vi "Create comm references.vi"() -> (0 "error out":errorcluster)   [LabVIEW 2019, in "Shared.lvlib"]
uses:
  Shared.lvlib
  Intertarget communication/Command + data + response cluster.ctl
  Intertarget communication/Status + response + data cluster.ctl
  Data message cluster.ctl
  mmWave data_class/mmWave data.lvclass
  Error event data.ctl
  Comm GV.vi
  Intertarget communication/CommandResponse communication.lvlib
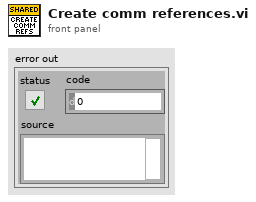
[diagram p1: front panel]
types:
  T1 = typedef "Shared.lvlib/Error event data.ctl" = cluster{"module":string, "info":string, "error":cluster{"Boolean Round":bool, "code":i32, "source":string}}
  T2 = typedef "Shared.lvlib/Data message cluster.ctl" = cluster{"group  ":string, "Data":refnum<class "mmWave data.lvclass">}
  T3 = typedef "CommandResponse communication.lvlib/Command + data + response cluster.ctl" = cluster{"message":string, "parameters":string, "response notifier":refnum<notifier>, "data":variant}
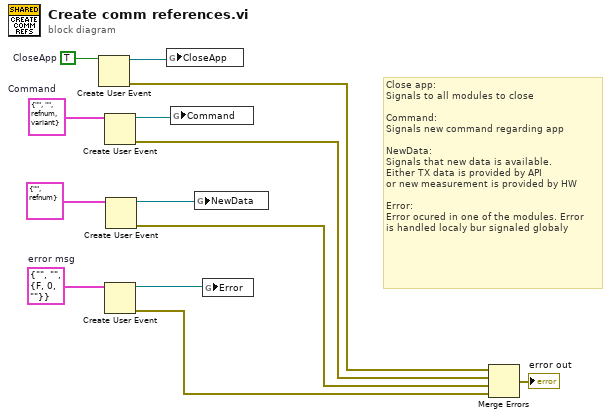
[diagram p0: block diagram]
diagram:
  w10 = T1 {"module"="", "info"="", "error"={"Boolean Round"=FALSE, "code"=0, "source"=""}}  # error msg
  w12 = T3 {"message"="", "parameters"="", "response notifier"=refnum, "data"=variant}  # Command
  w13 = TRUE  # CloseApp
  # "Close app:\nSignals to all modules to close\n\nCommand:\nSignals new command regarding app\n\nNewData:\nSignals that new data is available.\nEither TX data is provided by API\nor new measurement is provided by HW\n\nError:\nError ocured in one of the modules. Error\nis handled localy bur signaled globaly"
  n1 = Create User Event(user event datatype=w13) -> (user event=w4:refnum<user-event>, error out=w9:errorcluster)  [unwired: 1 in]
  n2 = Create User Event(user event datatype=w12) -> (user event=w3:refnum<user-event>, error out=w8:errorcluster)  [unwired: 1 in]
  n3 = Create User Event(user event datatype=w10) -> (user event=w1:refnum<user-event>, error out=w6:errorcluster)  [unwired: 1 in]
  n4 = Create User Event(user event datatype=T2 {"group  "="", "Data"=refnum} ("New data message")) -> (user event=w2:refnum<user-event>, error out=w7:errorcluster)  [unwired: 1 in]
  n5 = global write "Comm GV.vi" "CloseApp"(w4) -> ()
  n6 = global write "Comm GV.vi" "Command"(w3) -> ()
  n7 = global write "Comm GV.vi" "NewData"(w2) -> ()
  n8 = global write "Comm GV.vi" "Error"(w1) -> ()
  n9 = Merge Errors(w9, w8, w7, w6) -> (→"error out":errorcluster)
